vi "HexapodMoveHardware.vi"(7 "xyzuvw":dbl[](array[numeric]), 8 "error in (no error)":errorcluster, 9 "Positions of Axes to move":dbl[](array[numeric]), 10 "Axes to move":string[](array[string]), 11 "C-887 in":refnum<class "C-887.lvclass">) -> (0 "error out":errorcluster, 2 "Connection":T1, 3 "Move possible":cluster{"status":bool, "message":string})   [LabVIEW 2020, in "C-887.lvclass"]
uses:
  C-887.lvclass
  C:/GEECS/Developers Version/source/Device Drivers/HexapodPI/HexapodPI.lvclass
  HexapodPI.lvclass/HexapodPI.ctl
  C-887.lvclass/C-887.ctl
  Read Settings.vi
  Read positioners.vi
  shared/CompressAndUpdate(Poly)/CompressAndUpdate(Numeric).vi
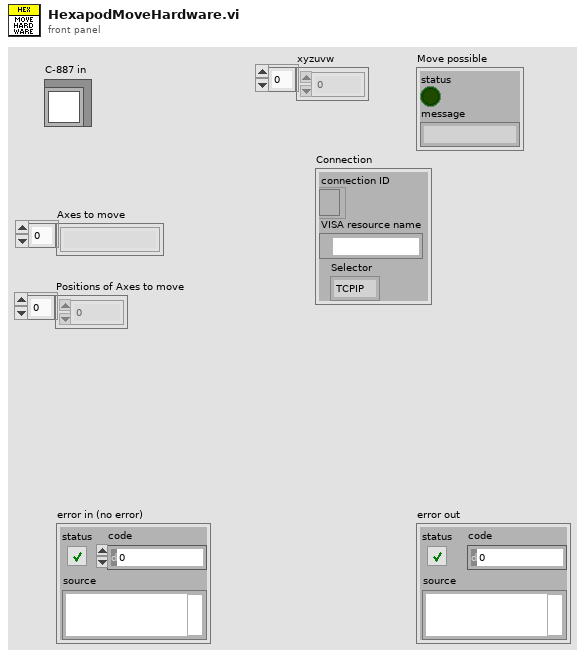
[diagram p1: front panel]
types:
  T1 = cluster{"connection ID":refnum<k5>, "VISA resource name":refnum<visa-resource-name>, "Selector":enum16{"TCPIP", "Serial"}}
  T2 = typedef "HexapodPI.lvclass/settingHexapod_TypDEf.ctl" = cluster{"xpos":cluster{"Value":dbl, "Min":dbl, "Max":dbl, "StepSize":dbl, "Tolerance":dbl, "ValueActual":dbl}, "ypos":cluster{"Value":dbl, "Min":dbl, "Max":dbl, "StepSize":dbl, "Tolerance":dbl, "ValueActual":dbl}, "zpos":cluster{"Value":dbl, "Min":dbl, "Max":dbl, "StepSize":dbl, "Tolerance":dbl, "ValueActual":dbl}, "uangle":cluster{"Value":dbl, "Min":dbl, "Max":dbl, "StepSize":dbl, "Tolerance":dbl, "ValueActual":dbl}, "vangle":cluster{"Value":dbl, "Min":dbl, "Max":dbl, "StepSize":dbl, "Tolerance":dbl, "ValueActual":dbl}, "devaddress":string, "connectiontype":enum16{"TCPIP", "Serial"}, "hexinit":enum16{"Not referenced", "Referenced"}, "status":enum16{"Not referenced", "Homing", "Moving", "Ready"}, "relativeMove":cluster{"Zpos":T3, "Zneg":T3, "Xpos":T3, "Xneg":T3, "Ypos":T3, "Yneg":T3, "Wpos":T3, "Wneg":T3, "Vpos":T3, "Vneg":T3, "Upos":T3, "Uneg":T3}, "stepsize":cluster{"Value":dbl, "Min":dbl, "Max":dbl, "StepSize":dbl, "Tolerance":dbl, "ValueActual":dbl}, "LaserAxis":cluster{"u":dbl, "v":dbl, "w":dbl}, "PivotPoint":T4, "wangle":cluster{"Value":dbl, "Min":dbl, "Max":dbl, "StepSize":dbl, "Tolerance":dbl, "ValueActual":dbl}, "LaserAxes":T3, "speed":cluster{"Value":dbl, "Min":dbl, "Max":dbl, "StepSize":dbl, "Tolerance":dbl, "ValueActual":dbl}, "Simulation":T3, "xyzuvw":dbl[], "xyzuvw_tolerances":dbl[]}
  T3 = typedef "OnOffTypeDef.ctl" = enum16{"off", "on"}
  T4 = typedef "PivotPoint_TypDef.ctl" = cluster{"R":cluster{"Value":dbl, "Min":dbl, "Max":dbl, "StepSize":dbl, "Tolerance":dbl, "ValueActual":dbl}, "S":cluster{"Value":dbl, "Min":dbl, "Max":dbl, "StepSize":dbl, "Tolerance":dbl, "ValueActual":dbl}, "T":cluster{"Value":dbl, "Min":dbl, "Max":dbl, "StepSize":dbl, "Tolerance":dbl, "ValueActual":dbl}}
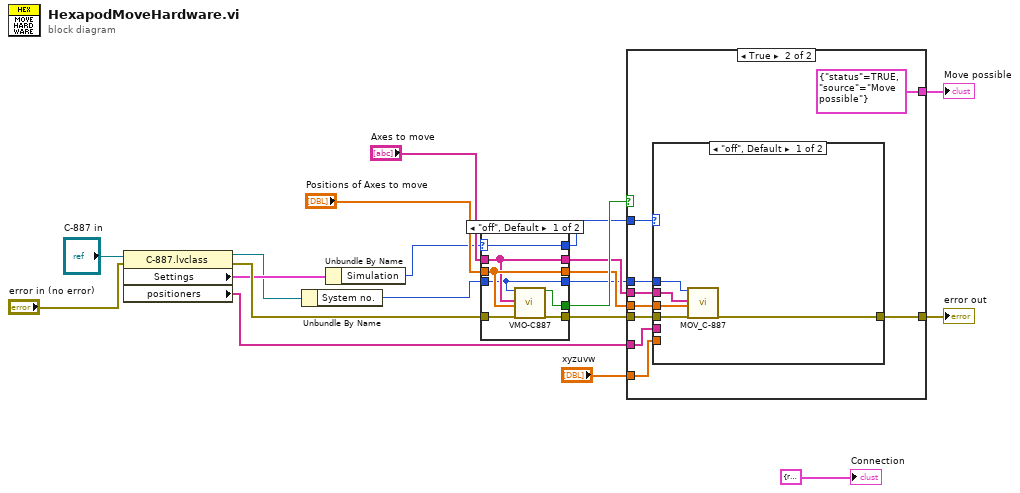
[diagram p0: block diagram]
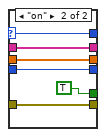
[diagram p2: hidden frame]
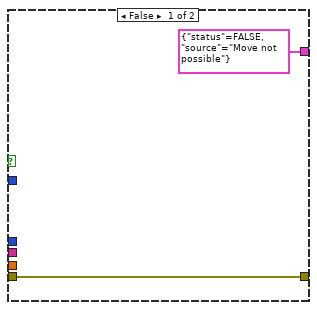
[diagram p3: hidden frame]
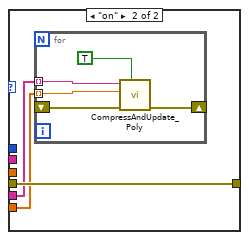
[diagram p4: hidden frame]
diagram:
  n1 = property class="C-887.lvclass"(reference="C-887 in", error in="error in (no error)") -> (reference out=w4:refnum<class "C-887.lvclass">, error out=w8:errorcluster, "Settings"=w6:T2, "positioners"=w7:string[])
  n2 = Unbundle By Name(w4) -> ("System no."=w3:i32)
  n3 = Unbundle By Name(w6) -> ("Simulation"=w5:T3)
  n4 = case shown="\"off\", Default" w5 {
    selector: w5 -> [w27 w29]
    tunnel: w8 -> [w26 w32]
    tunnel: "Positions of Axes to move" -> [w23 w30]
    tunnel: "Axes to move" -> [w22 w31]
    tunnel: [w25 w32] -> w17
    tunnel: [w24 TRUE ("Move possible")] -> w19
    tunnel: [w22 w31] -> w13
    tunnel: [w23 w30] -> w12
    tunnel: [w27 w29] -> w11
    tunnel: w3 -> [w21 w28]
    tunnel: [w21 w28] -> w2
    frame "off", Default {
      n5 = call "VMO-C887.vi"("System no."=w21, "Axes to command"=w22, "Position values"=w23, "error in"=w26) -> ("Move possible"=w24:bool, "error out"=w25:errorcluster)  [unwired: 14 in]
    }
    frame "on" {
    }
  }
  n6 = case shown="True" w19 {
    tunnel: w17 -> [w35 w44]
    tunnel: [w35 w43] -> w14
    tunnel: w13 -> [_ w42]
    tunnel: w12 -> [_ w41]
    tunnel: [cluster{"status":bool, "source":string} {"status"=FALSE, "source"="Move not possible"} ("error out") cluster{"status":bool, "source":string} {"status"=TRUE, "source"="Move possible"} ("error out")] -> w18
    tunnel: w11 -> [_ w39]
    tunnel: w7 -> [_ w38]
    tunnel: "xyzuvw" -> [_ w37]
    tunnel: w2 -> [_ w36]
    frame False {
    }
    frame True {
      n7 = case shown="\"off\", Default" w39 {
        tunnel: w44 -> [w49 w52]
        tunnel: [w48 w52] -> w43
        tunnel: w42 -> [w46 _]
        tunnel: w41 -> [w45 _]
        tunnel: w38 -> [_ w51]
        tunnel: w37 -> [_ w50]
        tunnel: w36 -> [w47 _]
        frame "off", Default {
          n8 = call "MOV_C-887.vi"("System no."=w47, "Axes to move"=w46, "Position values"=w45, "error in"=w49) -> ("error out"=w48:errorcluster)  [unwired: 15 in]
        }
        frame "on" {
          n9 = for {
            tunnel: w51 -> [w54] mode=indexing
            shift-right: [w57] -> _
            shift-left: _ -> [w55]
            tunnel: w50 -> [w53] mode=indexing
            n10 = call-poly "CompressAndUpdate_Poly.vi"("force CVT update (false)"=TRUE, "error in"=w55, "Numeric"=w53, "command or variable name"=w54) -> ("error out"=w57:errorcluster)  [unwired: 7 in]
          }
        }
      }
    }
  }
  "Move possible" <- w18
  "error out" <- w14
  "Connection" <- T1 {"connection ID"=refnum, "VISA resource name"="", "Selector"=enum."TCPIP"} ("Connection 2")
